vi "Format Input Channel List.vi"() -> (0 "Input Channels":string)   [LabVIEW 2013]
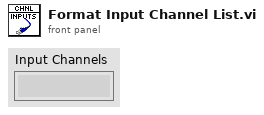
[diagram p1: front panel]
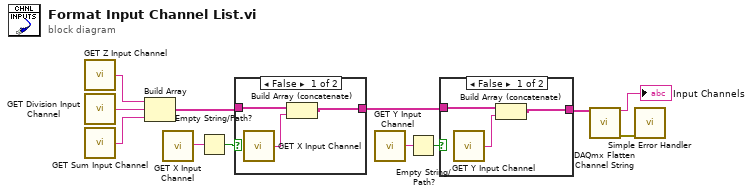
[diagram p0: block diagram]
diagram:
  n1 = call "GET Z Input Channel.vi"() -> ("Z Input Channel"=w9:string)
  n2 = call "GET Division Input Channel.vi"() -> ("Division Input Channel"=w10:string)
  n3 = call "GET Sum Input Channel.vi"() -> ("Sum Input Channel"=w11:string)
  n4 = Build Array(w9, w10, w11) -> (w4:string[])
  n5 = call "GET X Input Channel.vi"() -> ("X Input Channel"=w7:string)
  n6 = Empty String/Path?(string/path=w7) -> (empty?=w8:bool)
  n7 = case shown="False" w8 {
    tunnel: w4 -> [w14 w16]
    tunnel: [w15 w16] -> w12
    frame False {
      n8 = call "GET X Input Channel.vi"() -> ("X Input Channel"=w13:string)
      n9 = Build Array (concatenate)(w14, w13) -> (w15:string[])
    }
    frame True {
    }
  }
  n10 = call "GET Y Input Channel.vi"() -> ("Y Input Channel"=w5:string)
  n11 = Empty String/Path?(string/path=w5) -> (empty?=w6:bool)
  n12 = case shown="False" w6 {
    tunnel: w12 -> [w18 w20]
    tunnel: [w19 w20] -> w3
    frame False {
      n13 = call "GET Y Input Channel.vi"() -> ("Y Input Channel"=w17:string)
      n14 = Build Array (concatenate)(w18, w17) -> (w19:string[])
    }
    frame True {
    }
  }
  n15 = call <vilib>:"DAQmx Flatten Channel String.vi"("names in"=w3) -> ("names out"=→"Input Channels":string, "error out"=w1:errorcluster)  [unwired: 13 in]
  n16 = call <vilib>:"Simple Error Handler.vi"("error in (no error)"=w1) -> ()  [unwired: 4 in, 5 out]
